vi "Create DataSet by Name.vi"(8 "错误输入（无错误）":errorcluster, 11 "dataSetName":string) -> (0 "错误输出":errorcluster, 3 "DataSet Out":refnum<k24>)   [LabVIEW 2012, in "DataGridView.lvlib"]
uses:
  DataGridView.lvlib
  System.Data
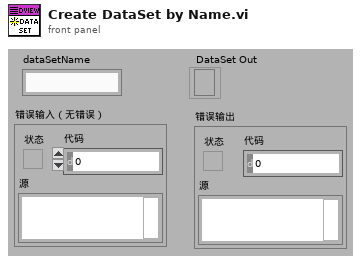
[diagram p1: front panel]
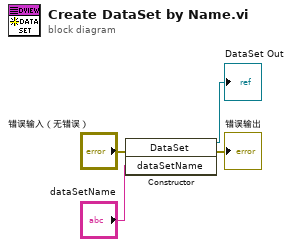
[diagram p0: block diagram]
diagram:
  n1 = constructor class="DataSet"(error in="错误输入（无错误）", "dataSetName"="dataSetName") -> (reference out=→"DataSet Out":refnum<k24>, error out=→"错误输出":errorcluster)  [unwired: 2 in, 2 out]
